vi "fakeLineCreation.vi"(8 "volume info":T2, 9 "ch1":bool[](array[boolean]), 10 "ch0":bool[](array[boolean]), 11 "voxel number":u32) -> (0 "line":T1, 1 "ch1 out":bool[](array[boolean]), 2 "ch0 out":bool[](array[boolean]), 3 "voxel number out":u32)   [LabVIEW 2010]
panel:
  out "zi":u32
  out "xi":u32
  out "yi":u32
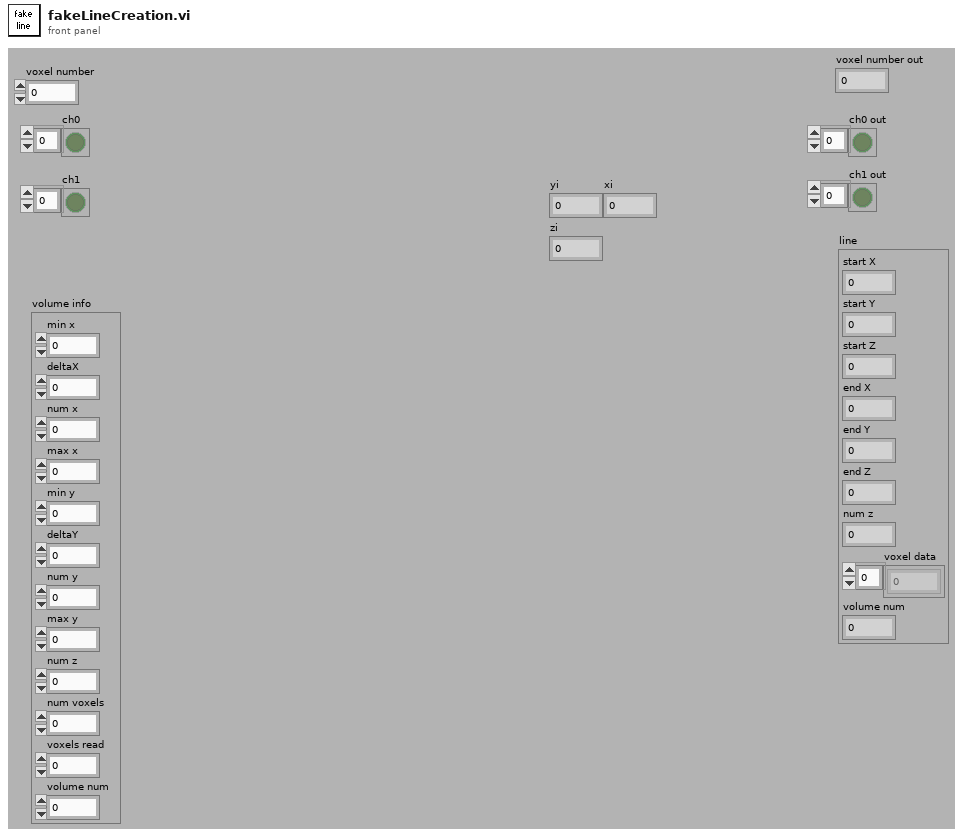
[diagram p1: front panel]
types:
  T1 = cluster{"start X":i16, "start Y":i16, "start Z":i16, "end X":i16, "end Y":i16, "end Z":i16, "num z":u8, "voxel data":u32[], "volume num":u32}
  T2 = cluster{"min x":i16, "deltaX":dbl, "num x":u32, "max x":i16, "min y":i16, "deltaY":dbl, "num y":u32, "max y":i16, "num z":u32, "num voxels":u32, "voxels read":u32, "volume num":u32}
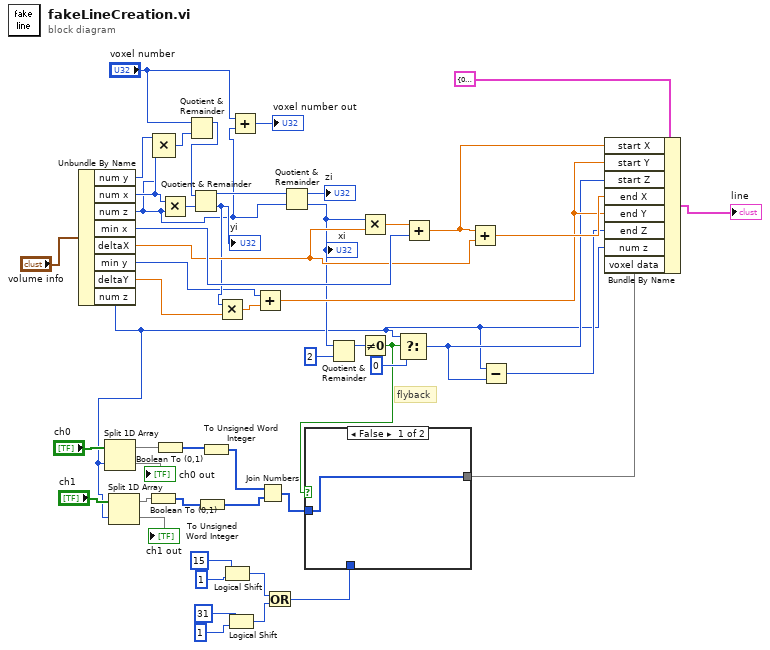
[diagram p0: block diagram]
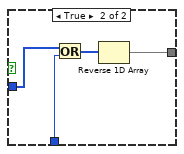
[diagram p2: hidden frame]
diagram:
  # "flyback"
  n1 = Unbundle By Name("volume info") -> ("num y"=w10:u32, "num x"=w9:u32, "num z"=w8:u32, "min x"=w44:i16, "deltaX"=w42:dbl, "min y"=w37:i16, "deltaY"=w39:dbl, "num z"=w12:u32)
  n2 = Split 1D Array(array="ch0", index=w12) -> (first subarray=w18:bool[], second subarray=→"ch0 out":bool[])
  n3 = Split 1D Array(array="ch1", index=w12) -> (first subarray=w16:bool[], second subarray=→"ch1 out":bool[])
  n4 = Boolean To (0,1)(Boolean=w16) -> (0, 1=w27:i16[])
  n5 = Compound Arithmetic op=MULTIPLY(w10, w9, w8) -> (w6:u32)
  n6 = Boolean To (0,1)(Boolean=w18) -> (0, 1=w28:i16[])
  n7 = Multiply(x=w9, y=w8) -> (x*y=w48:u32)
  n8 = Quotient & Remainder(x="voxel number", y=w6) -> (x-y*floor(x/y)=w7:u32)  [unwired: 1 out]
  n9 = Quotient & Remainder(x=w7, y=w48) -> (x-y*floor(x/y)=w47:u32, floor(x/y)=w40:u32)
  "yi" <- w40
  n10 = To Unsigned Word Integer(number=w27) -> (unsigned 16bit integer=w25:u16[])
  n11 = To Unsigned Word Integer(number=w28) -> (unsigned 16bit integer=w26:u16[])
  n12 = Multiply(x=w40, y=w39) -> (x*y=w38:dbl)
  n13 = Logical Shift(y=i8 15, x=u32 1) -> (x << y=w20:u32)
  n14 = Logical Shift(y=i8 31, x=u32 1) -> (x << y=w19:u32)
  n15 = Add(x="voxel number", y=w8) -> (x+y=→"voxel number out":u32)
  n16 = Add(x=w37, y=w38) -> (x+y=w36:dbl)
  n17 = Join Numbers(hi=w26, lo=w25) -> ((hi.lo)=w4:u32[])
  n18 = Or(x=w20, y=w19) -> (x .or. y?=w3:u32)
  n19 = Quotient & Remainder(x=w47, y=w8) -> (x-y*floor(x/y)=→"zi":u32, floor(x/y)=w35:u32)
  "xi" <- w35
  n20 = Quotient & Remainder(x=w35, y=u32 2) -> (x-y*floor(x/y)=w33:u32)  [unwired: 1 out]
  n21 = Multiply(x=w35, y=w42) -> (x*y=w45:dbl)
  n22 = Not Equal To 0?(x=w33) -> (x != 0?=w5:bool)
  n23 = case shown="False" w5 {
    tunnel: w4 -> [w51 w55]
    tunnel: w3 -> [_ w54]
    tunnel: [w51 w52] -> w2
    frame False {
    }
    frame True {
      n24 = Or(x=w55, y=w54) -> (x .or. y?=w53:u32[])
      n25 = Reverse 1D Array(array=w53) -> (reversed array=w52:u32[])
    }
  }
  n26 = Select(t=w12, s=w5, f=u32 0) -> (s? t:f=w31:u32)
  n27 = Add(x=w45, y=w44) -> (x+y=w43:dbl)
  n28 = Add(x=w43, y=w42) -> (x+y=w41:dbl)
  n29 = Subtract(x=w12, y=w31) -> (x-y=w30:u32)
  n30 = Bundle By Name(cluster=T1 {"start X"=0, "start Y"=0, "start Z"=0, "end X"=0, "end Y"=0, "end Z"=0, "num z"=0, "voxel data"=[], "volume num"=0} ("line"), "start X"=w43, "start Y"=w36, "start Z"=w31, "end X"=w41, "end Y"=w36, "end Z"=w30, "num z"=w12, "voxel data"=w2) -> (→"line":T1)
